vi "Get All First Level Nodes With Children.vi"(8 "error in":errorcluster, 11 "Fast Tree in":refnum<class "Fast Tree.lvclass">) -> (0 "error out":errorcluster, 2 "Top Level With Children":T1(array[cluster]), 3 "Fast Tree out":refnum<class "Fast Tree.lvclass">)   [LabVIEW 2019, in "Fast Tree.lvclass"]
uses:
  Fast Tree.lvclass
  Fast Tree.lvclass/Fast Tree.ctl
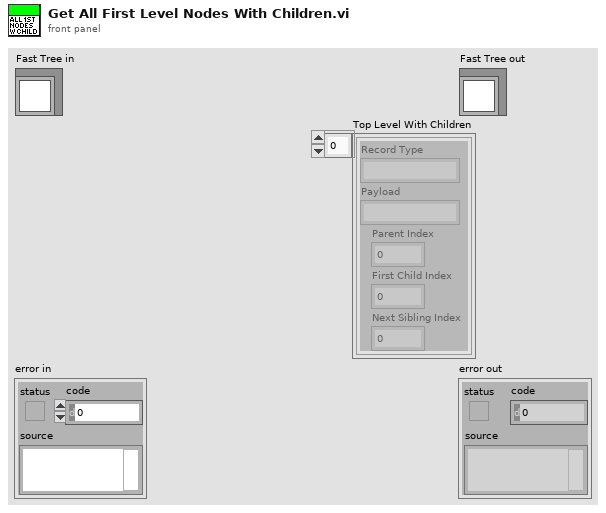
[diagram p1: front panel]
types:
  T1 = cluster{"Record Type":string, "Payload":string, "Parent Index":i32, "First Child Index":i32, "Next Sibling Index":i32}[]
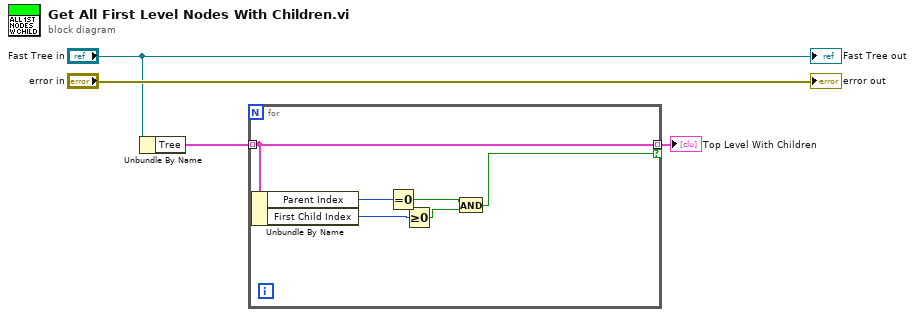
[diagram p0: block diagram]
diagram:
  n1 = Unbundle By Name("Fast Tree in") -> ("Tree"=w2:T1)
  n2 = for {
    tunnel: w2 -> [w6] mode=indexing
    tunnel: [w6] -> w1 mode=indexing if=w5
    n3 = Unbundle By Name(w6) -> ("Parent Index"=w10:i32, "First Child Index"=w9:i32)
    n4 = Equal To 0?(x=w10) -> (x = 0?=w8:bool)
    n5 = Greater Or Equal To 0?(x=w9) -> (x >= 0?=w7:bool)
    n6 = And(x=w8, y=w7) -> (x .and. y?=w5:bool)
  }
  "Top Level With Children" <- w1
  "error out" <- "error in"
  "Fast Tree out" <- "Fast Tree in"
